vi "Step control.vi"(8 "error in":errorcluster) -> (0 "error out":errorcluster, 3 "Step elapsed time,  s":u32)   [LabVIEW 2014]
uses:
  Control/Sub step profiler.ctl
  Control/Step name enum.ctl
  Step global.vi
  <vilib>/Automated Test Systems Ltd/General Tools/Stopwatch/Stop watch/Stop watch.lvlib
panel:
  in  "Step cluster":T2={"Step number"=0, "Step Name"="", "Step name enum"=enum."Init NI", "Start condition 1 name"="", "Start condition 1 comparator"="", "Start condition 1 value"=0.0, "Start condition 2 name"="", "Start condition 2 comparator"="", "Start condition 2 value"=0.0, "Start condition 3 name"="", "Start condition 3 comparator"="", "Start condition 3 value"=0.0, "End condition 1 name"="", "End condition 1 comparator"="", "End condition 1 value"=0.0, "End condition 2 name"="", "End condition 2 comparator"="", "End condition 2 value"=0.0, "End condition 3 name"="", "End condition 3 comparator"="", "End condition 3 value"=0.0, "Constant condition 1 name"="", "Constant condition 1 comparator"="", "Constant condition 1 value"=0.0, "Constant condition 2 name"="", "Constant condition 2 comparator"="", "Constant condition 2 value"=0.0, "Constant condition 3 name"="", "Constant condition 3 comparator"="", "Constant condition 3 value"=0.0, "Duration, mS"=0.0, "Max Duration, mS"=0.0}
  in  "Sub step":T3
  out "Step Name":string
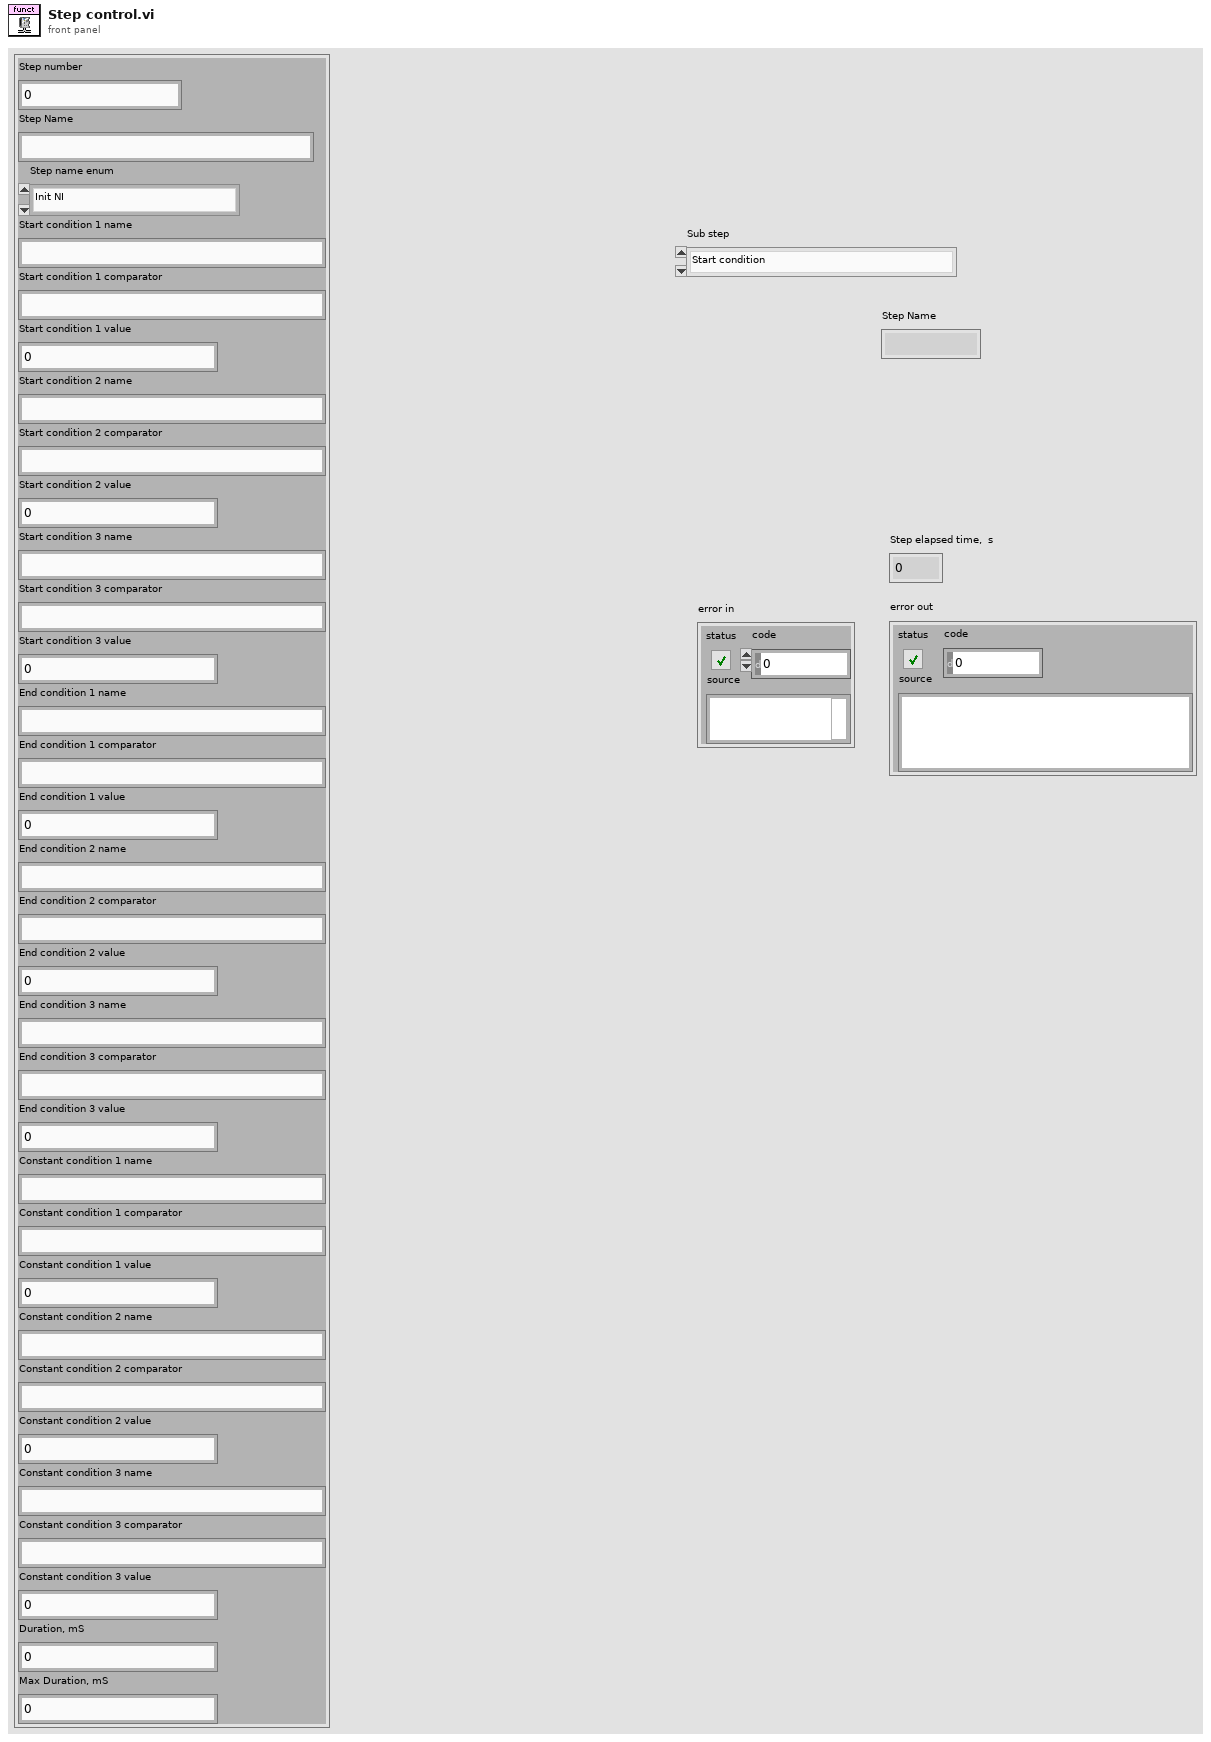
[diagram p1: front panel]
types:
  T1 = typedef "Step name enum.ctl" = enum16{"Default", "Idle", "Init Ard", "Init SM", "Init NI", "Run", "Close"}
  T2 = cluster{"Step number":i32, "Step Name":string, "Step name enum":T1, "Start condition 1 name":string, "Start condition 1 comparator":string, "Start condition 1 value":dbl, "Start condition 2 name":string, "Start condition 2 comparator":string, "Start condition 2 value":dbl, "Start condition 3 name":string, "Start condition 3 comparator":string, "Start condition 3 value":dbl, "End condition 1 name":string, "End condition 1 comparator":string, "End condition 1 value":dbl, "End condition 2 name":string, "End condition 2 comparator":string, "End condition 2 value":dbl, "End condition 3 name":string, "End condition 3 comparator":string, "End condition 3 value":dbl, "Constant condition 1 name":string, "Constant condition 1 comparator":string, "Constant condition 1 value":dbl, "Constant condition 2 name":string, "Constant condition 2 comparator":string, "Constant condition 2 value":dbl, "Constant condition 3 name":string, "Constant condition 3 comparator":string, "Constant condition 3 value":dbl, "Duration, mS":dbl, "Max Duration, mS":dbl}
  T3 = typedef "Sub step profiler.ctl" = enum16{"Start condition", "Constant condition", "End condition", "Fail", "Complete"}
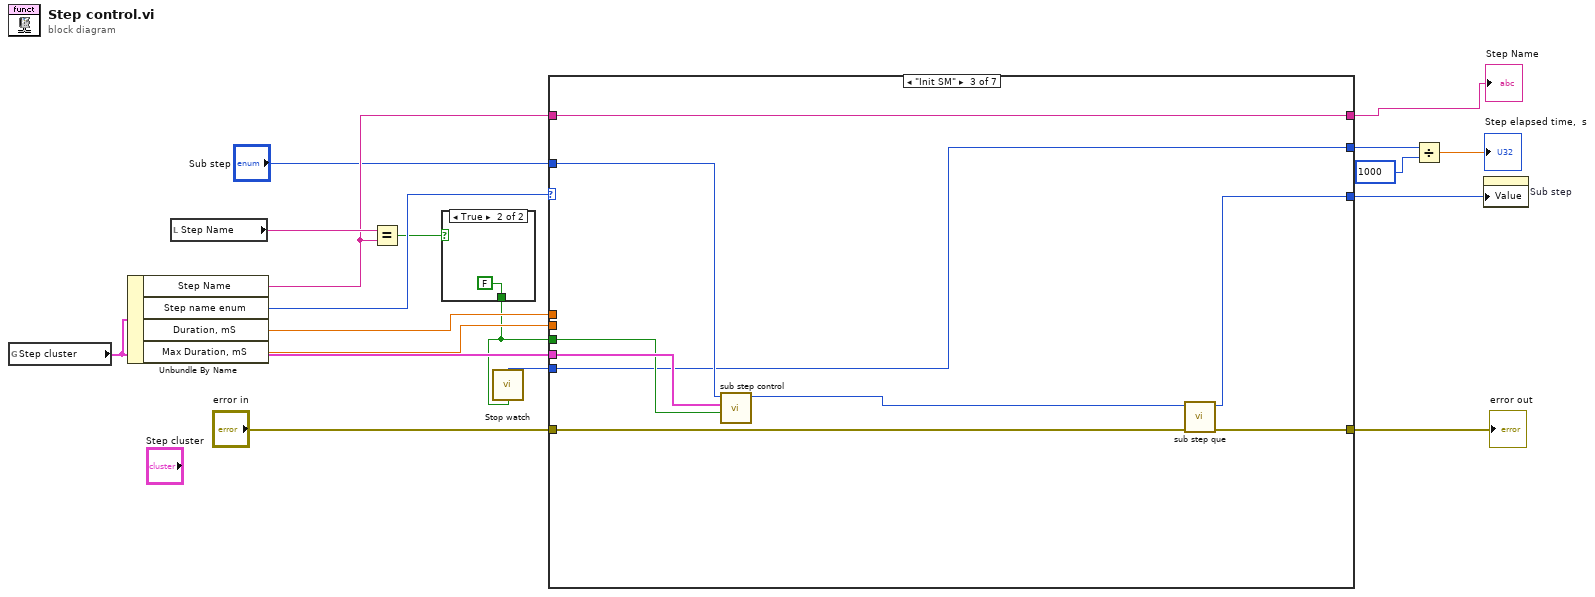
[diagram p0: block diagram]
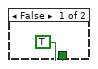
[diagram p2: hidden frame]
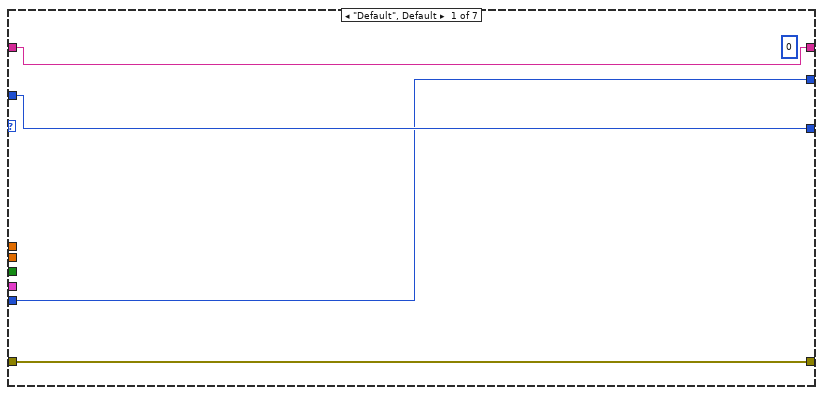
[diagram p3: hidden frame]
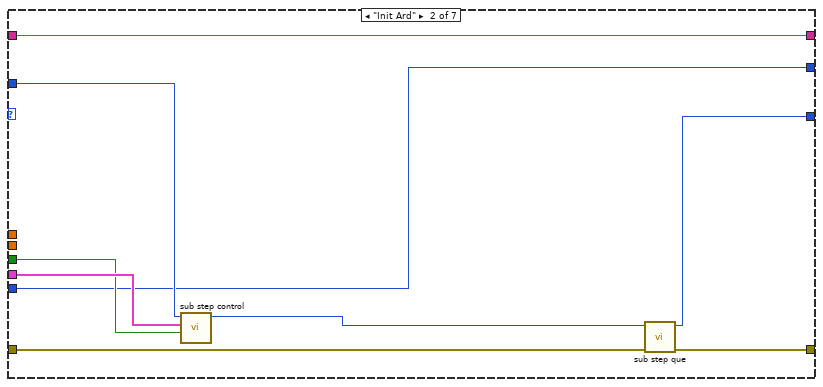
[diagram p4: hidden frame]
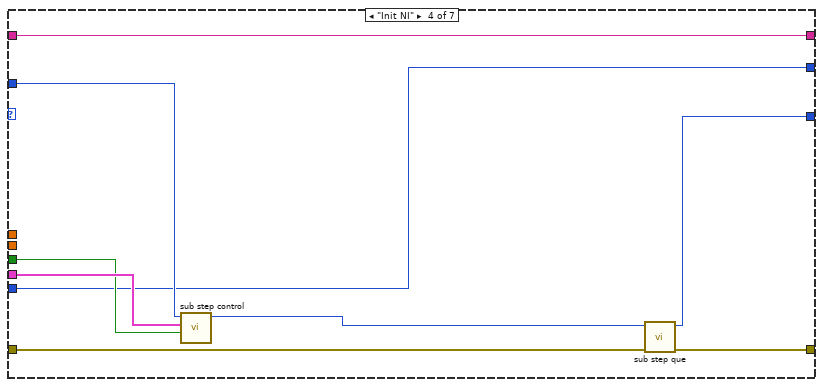
[diagram p5: hidden frame]
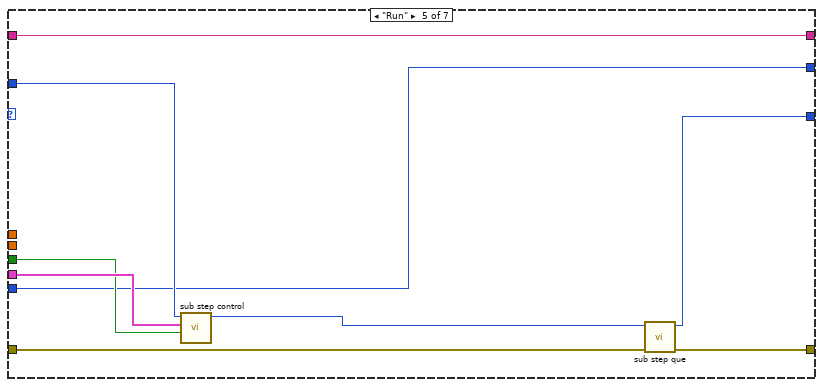
[diagram p6: hidden frame]
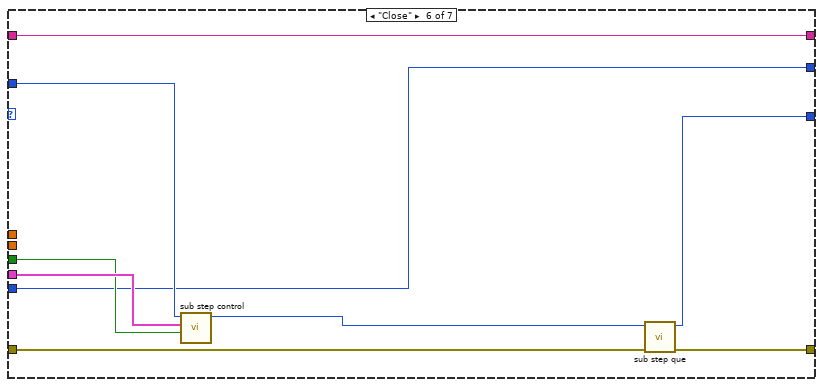
[diagram p7: hidden frame]
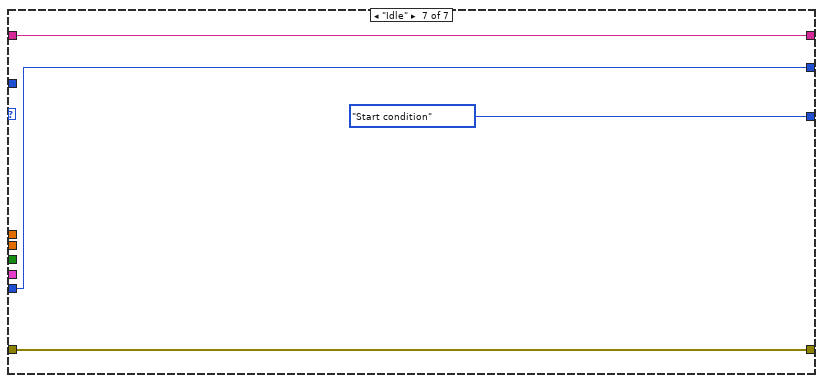
[diagram p8: hidden frame]
diagram:
  n1 = global read "Step global.vi" "Step cluster"() -> (w16:T2)
  n2 = Unbundle By Name(w16) -> ("Step Name"=w8:string, "Step name enum"=w12:T1, "Duration, mS"=w6:dbl, "Max Duration, mS"=w2:dbl)
  n3 = local read "Step Name"() -> (w9:string)
  n4 = Equal?(x=w9, y=w8) -> (x = y?=w10:bool)
  n5 = case shown="True" w10 {
    tunnel: [TRUE FALSE] -> w1
    frame False {
    }
    frame True {
    }
  }
  n6 = call <vilib>:"Stop watch.vi"("reset timer"=w1) -> ("Elapsed time, ms"=w3:u32)  [unwired: 13 in, 1 out]
  n7 = case shown="\"Init SM\"" w12 {
    tunnel: [w23 w26 w35 w44 w53 w62 w72] -> w17
    tunnel: "error in" -> [w23 w27 w36 w45 w54 w63 w72]
    tunnel: w16 -> [_ w31 w40 w49 w58 w67 _]
    tunnel: w8 -> [w22 w32 w41 w50 w59 w68 w71]
    tunnel: [w20 w28 w37 w46 w55 w64 w69] -> w15
    tunnel: w1 -> [_ w29 w38 w47 w56 w65 _]
    tunnel: [w22 w32 w41 w50 w59 w68 w71] -> w7
    tunnel: w6 -> [_ _ _ _ _ _ _]
    tunnel: w2 -> [_ _ _ _ _ _ _]
    tunnel: [w21 w24 w33 w42 w51 w60 Sub_step_profiler."Start condition" ("Sub step")] -> w4
    tunnel: "Sub step" -> [w21 w30 w39 w48 w57 w66 _]
    tunnel: w3 -> [w20 w28 w37 w46 w55 w64 w69]
    frame "Default", Default {
      (unwired) 0
    }
    frame "Init Ard" {
      n8 = call "sub step control.vi"("First time?"=w29, "Step cluster"=w31, "Sub step"=w30) -> ("Sub step out"=w25:T3)  [unwired: 8 in]
      n9 = call "sub step que.vi"("error in"=w27, "Sub step in"=w25) -> ("error out"=w26:errorcluster, "Sub step out"=w24:T3)  [unwired: 8 in]
    }
    frame "Init SM" {
      n10 = call "sub step control.vi"("First time?"=w38, "Step cluster"=w40, "Sub step"=w39) -> ("Sub step out"=w34:T3)  [unwired: 8 in]
      n11 = call "sub step que.vi"("error in"=w36, "Sub step in"=w34) -> ("error out"=w35:errorcluster, "Sub step out"=w33:T3)  [unwired: 8 in]
    }
    frame "Init NI" {
      n12 = call "sub step control.vi"("First time?"=w47, "Step cluster"=w49, "Sub step"=w48) -> ("Sub step out"=w43:T3)  [unwired: 8 in]
      n13 = call "sub step que.vi"("error in"=w45, "Sub step in"=w43) -> ("error out"=w44:errorcluster, "Sub step out"=w42:T3)  [unwired: 8 in]
    }
    frame "Run" {
      n14 = call "sub step control.vi"("First time?"=w56, "Step cluster"=w58, "Sub step"=w57) -> ("Sub step out"=w52:T3)  [unwired: 8 in]
      n15 = call "sub step que.vi"("error in"=w54, "Sub step in"=w52) -> ("error out"=w53:errorcluster, "Sub step out"=w51:T3)  [unwired: 8 in]
    }
    frame "Close" {
      n16 = call "sub step control.vi"("First time?"=w65, "Step cluster"=w67, "Sub step"=w66) -> ("Sub step out"=w61:T3)  [unwired: 8 in]
      n17 = call "sub step que.vi"("error in"=w63, "Sub step in"=w61) -> ("error out"=w62:errorcluster, "Sub step out"=w60:T3)  [unwired: 8 in]
    }
    frame "Idle" {
    }
  }
  "error out" <- w17
  "Step Name" <- w7
  n18 = Divide(x=w15, y=u32 1000 ("x")) -> (x/y=→"Step elapsed time,  s":dbl)
  n19 = property on="Sub step" class="Enum (strict)"("Value"=w4) -> ()  [unwired: 2 in, 2 out]
